vi "SPM Pump v0.5.vi"(0 "Termination char\n(0xA = '\\n' = LF)\n(0xD = '\\r' = CR)":u8=13 format="%.0x", 1 "Enable Termination\nChar (T)":bool=TRUE, 2 "Timeout (ms)":u32=10000, 3 "Serial Settings:Serial End Mode for Reads":u16(ring)=2 items=["None", "LastBit", "TermChar"], 4 "byte count":u32=64, 5 "Delay before read (ms)":u32=1000, 6 "Time <input>":dbl, 7 "error in (no error)":errorcluster, 8 "Serial port input":string="/1ZR", 9 "VISA resource name":refnum<visa-resource-name>="COM6", 10 "parity":u16(ring) items=["None", "Odd", "Even", "Mark", "Space"], 11 "baud rate":u32=9600, 12 "stop bits":u16(ring)=10 items=["1.0"=10, "1.5"=15, "2.0"=20], 13 "data bits":u16=8 min=5 max=8 step=1, 14 "flow control":u16(ring) items=["None"=0, "XON/XOFF"=1, "RTS/CTS"=2, "DTR/DSR"=4], 15 "Time units <input>":string) -> (16 "Input command":string, 18 "Pump status":string, 20 "Start speed":i32, 21 "Maximal speed":i32, 22 "Cutoff speed":i32, 23 "Valve position":i32, 24 "Absolute plunger position":i32, 25 "Actual plunger position":i32, 26 "Serial port":string, 27 "error out":errorcluster)   [LabVIEW 2016]
doc: "The Basic Serial Read and Write example performs a Serial Port Read, a Serial Port Write, or a combination of these actions. The user selects the actions (read or write) on the front panel. If both are selected, the VI will write the data first, read data, and then close the VISA session that is opened to the port. This VI will wait until the specified number of bytes is received at the port. Only the number of bytes specified will be read.\n\nINSTRUCTIONS:\n1) Select the serial resource and configuration parameters (baud rate, data bits, parity, stop bits, flow control).\n2) Select the operations to be performed. \n3) Connect the serial port to your device. If no device is available, perform a loopback test by doing one of the following. Short pins 2 and 3 on a RS-232 cable or short pin 4 to pin 8 and pin 5 to pin 9 on a RS-485/422 cable. \n4) Run the VI to see the data read. (The \"read string\" will match the \"string to write\" if a loopback test was performed.)\n\nNote: The parameters set for the serial port must match the parameters of the connected instrument or device. In this example, the bytes to read parameter specifies the number of bytes that the serial port reads. If there were more bytes at the port than the number specified in bytes to read, those bytes would not be read. Also, if you specify to read more bytes than the number of bytes actually read, you might receive a timeout error message.\n\nOn the block diagram, the Configure Serial Port VI sets the configuration parameters. The front panel displays the controls used to configure the basic parameters, such as baud rate, data bits, and parity. Constants configure the other parameters the user probably does not need set. After the VISA Configure Serial Port VI opens the VISA session and configures the port, the VI passes the VISA resource name to other VIs that perform operations on that VISA resource. The VISA Write function sends a command to the serial device and the VISA Read function returns data based on the command. The VISA Close function then closes the reference to the serial device. It is important to close the reference; otherwise communication through with that port through protocols other than VISA might not be possible."
panel:
  # "Select the serial resource and the operations (Read, Write, or both) to be performed.  If both are selected, the VI will write the data first, read data and then close the VISA session that is opened to the port.  This VI will wait until the specified number of bytes is received at the port. Only the number of bytes specified will be read."
  # "For additional information select File >> VI Properties >> Documentation"
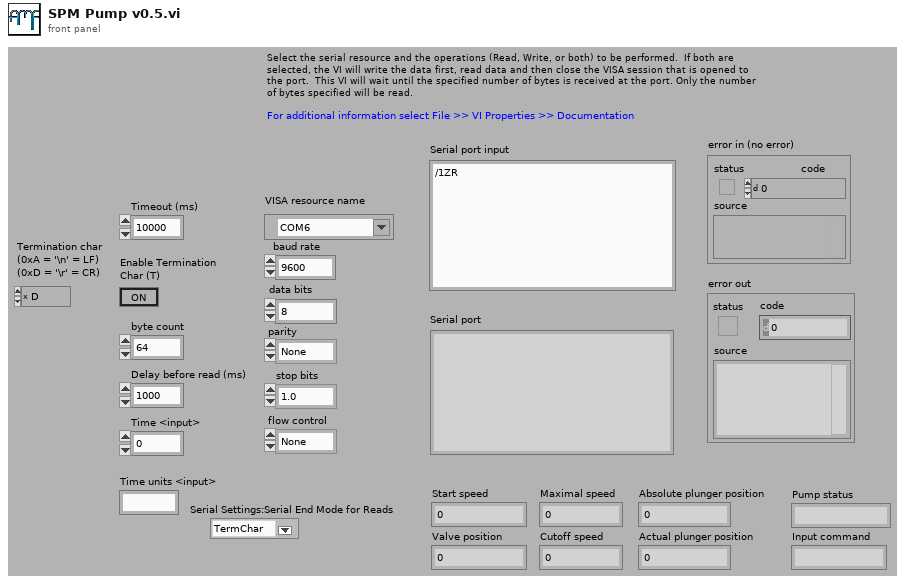
[diagram p1: front panel]
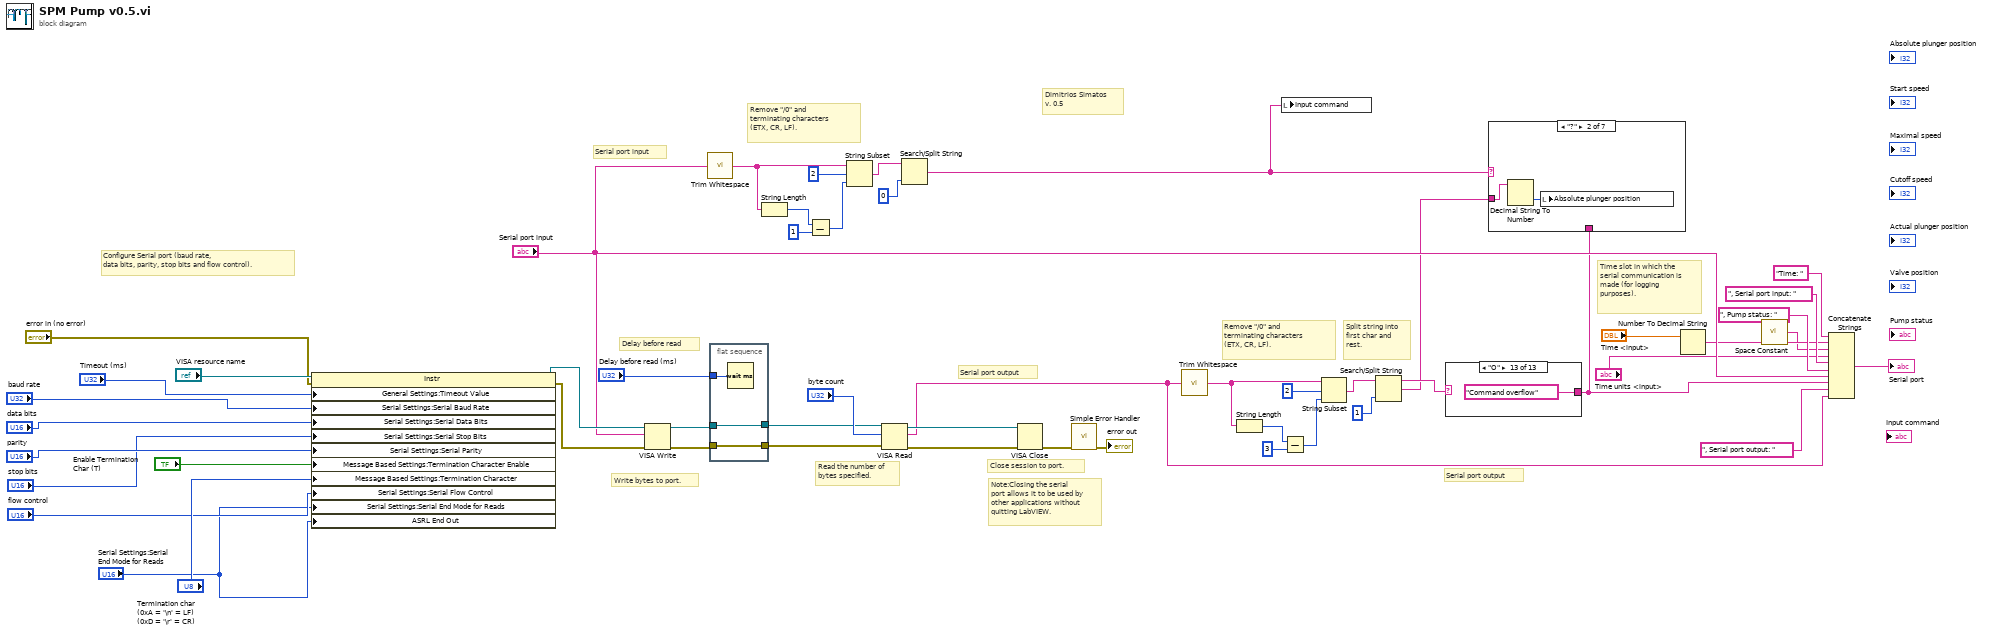
[diagram p0: block diagram]
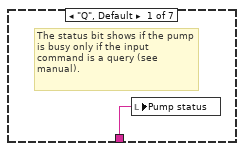
[diagram p2: hidden frame]
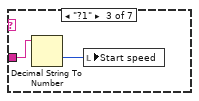
[diagram p3: hidden frame]
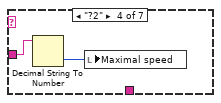
[diagram p4: hidden frame]
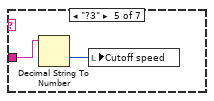
[diagram p5: hidden frame]
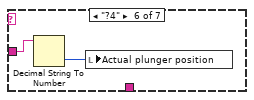
[diagram p6: hidden frame]
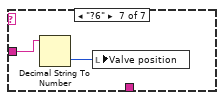
[diagram p7: hidden frame]
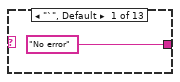
[diagram p8: hidden frame]
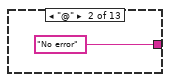
[diagram p9: hidden frame]
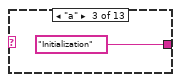
[diagram p10: hidden frame]
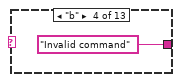
[diagram p11: hidden frame]
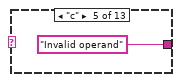
[diagram p12: hidden frame]
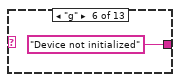
[diagram p13: hidden frame]
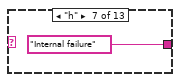
[diagram p14: hidden frame]
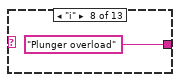
[diagram p15: hidden frame]
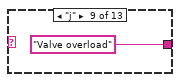
[diagram p16: hidden frame]
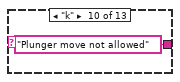
[diagram p17: hidden frame]
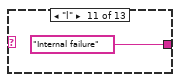
[diagram p18: hidden frame]
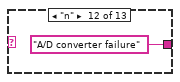
[diagram p19: hidden frame]
diagram:
  # "Serial port input"
  # "Remove \"/0\" and terminating characters (ETX, CR, LF)."
  # "Serial port output"
  # "Serial port output"
  # "Time slot in which the serial communication is made (for logging purposes)."
  # "Split string into first char and rest."
  # "Remove \"/0\" and terminating characters (ETX, CR, LF)."
  # "Delay before read"
  # "Dimitrios Simatos\nv. 0.5"
  # "Read the number of bytes specified."
  # "Write bytes to port."
  # "Note:Closing the serial port allows it to be used by other applications without\nquitting LabVIEW."
  # "Configure Serial port (baud rate,\ndata bits, parity, stop bits and flow control)."
  # "Close session to port."
  n1 = property class="Instr"(reference="VISA resource name", error in="error in (no error)", "General Settings:Timeout Value"="Timeout (ms)", "Serial Settings:Serial Baud Rate"="baud rate", "Serial Settings:Serial Data Bits"="data bits", "Serial Settings:Serial Stop Bits"="stop bits", "Serial Settings:Serial Parity"="parity", "Message Based Settings:Termination Character Enable"="Enable Termination\nChar (T)", "Message Based Settings:Termination Character"="Termination char\n(0xA = '\\n' = LF)\n(0xD = '\\r' = CR)", "Serial Settings:Serial Flow Control"="flow control", "Serial Settings:Serial End Mode for Reads"="Serial Settings:Serial End Mode for Reads", "ASRL End Out"="Serial Settings:Serial End Mode for Reads") -> (reference out=w39:refnum<visa-resource-name>, error out=w38:errorcluster)
  n2 = VISA Write(VISA resource name=w39, write buffer="Serial port input", error in (no error)=w38) -> (VISA resource name out=w34:refnum<visa-resource-name>, error out=w33:errorcluster)  [unwired: 1 out]
  n3 = call <vilib>:"Trim Whitespace.vi"("string"="Serial port input") -> ("trimmed string"=w12:string)  [unwired: 1 in]
  n4 = flat-sequence {
    tunnel: w33 -> [w54]
    tunnel: [w54] -> w32
    tunnel: w34 -> [w53]
    tunnel: [w53] -> w31
    tunnel: "Delay before read (ms)" -> [w55]
    frame #0 {
      n5 = Wait (ms)(milliseconds to wait=w55) -> ()  [unwired: 1 out]
    }
  }
  n6 = String Length(string=w12) -> (length=w16:i32)
  n7 = Subtract(x=w16, y=1) -> (x-y=w15:i32)
  n8 = String Subset(string=w12, offset (0)=2, length (rest)=w15) -> (substring=w9:string)
  n9 = VISA Read(VISA resource name=w31, byte count="byte count", error in (no error)=w32) -> (VISA resource name out=w51:refnum<visa-resource-name>, read buffer=w18:string, error out=w52:errorcluster)  [unwired: 1 out]
  n10 = Search/Split String(string=w9, offset (0)=0) -> (match + rest of string=w1:string)  [unwired: 1 in, 2 out]
  n11 = VISA Close(VISA resource name=w51, error in (no error)=w52) -> (error out=w50:errorcluster)
  n12 = call <vilib>:"Simple Error Handler.vi"("error in (no error)"=w50) -> ("error out"=→"error out":errorcluster)  [unwired: 4 in, 4 out]
  n13 = call <vilib>:"Trim Whitespace.vi"("string"=w18) -> ("trimmed string"=w25:string)  [unwired: 1 in]
  n14 = String Length(string=w25) -> (length=w29:i32)
  n15 = local write "Input command"(w1) -> ()
  n16 = Subtract(x=w29, y=3) -> (x-y=w28:i32)
  n17 = String Subset(string=w25, offset (0)=2, length (rest)=w28) -> (substring=w24:string)
  n18 = Search/Split String(string=w24, offset (0)=1) -> (substring before match=w22:string, match + rest of string=w8:string)  [unwired: 1 in, 1 out]
  n19 = case shown="\"O\"" w22 {
    tunnel: ["No error" "No error" "Initialization" "Invalid command" "Invalid operand" "Device not initialized" "Internal failure" "Plunger overload" "Valve overload" "Plunger move not allowed" "Internal failure" "A/D converter failure" "Command overflow"] -> w7
    frame "`", Default {
    }
    frame "@" {
    }
    frame "a" {
    }
    frame "b" {
    }
    frame "c" {
    }
    frame "g" {
    }
    frame "h" {
    }
    frame "i" {
    }
    frame "j" {
    }
    frame "k" {
    }
    frame "l" {
    }
    frame "n" {
    }
    frame "O" {
    }
  }
  n20 = case shown="\"?\"" w1 {
    tunnel: w8 -> [_ w70 w72 w75 w76 w79 w81]
    tunnel: w7 -> [w69 _ _ _ _ _ _]
    frame "Q", Default {
      # "The status bit shows if the pump is busy only if the input command is a query (see manual)."
      n21 = local write "Pump status"(w69) -> ()
    }
    frame "?" {
      n22 = Decimal String To Number(string=w70) -> (number=w71:i32)  [unwired: 2 in, 1 out]
      n23 = local write "Absolute plunger position"(w71) -> ()
    }
    frame "?1" {
      n24 = Decimal String To Number(string=w72) -> (number=w73:i32)  [unwired: 2 in, 1 out]
      n25 = local write "Start speed"(w73) -> ()
    }
    frame "?2" {
      n26 = Decimal String To Number(string=w75) -> (number=w74:i32)  [unwired: 2 in, 1 out]
      n27 = local write "Maximal speed"(w74) -> ()
    }
    frame "?3" {
      n28 = Decimal String To Number(string=w76) -> (number=w77:i32)  [unwired: 2 in, 1 out]
      n29 = local write "Cutoff speed"(w77) -> ()
    }
    frame "?4" {
      n30 = Decimal String To Number(string=w79) -> (number=w78:i32)  [unwired: 2 in, 1 out]
      n31 = local write "Actual plunger position"(w78) -> ()
    }
    frame "?6" {
      n32 = Decimal String To Number(string=w81) -> (number=w80:i32)  [unwired: 2 in, 1 out]
      n33 = local write "Valve position"(w80) -> ()
    }
  }
  n34 = Number To Decimal String(number="Time <input>") -> (decimal integer string=w4:string)  [unwired: 1 in]
  n35 = call <vilib>:"Space Constant.vi"() -> ("String"=w2:string)
  n36 = Concatenate Strings("Time: ", w4, w2, "Time units <input>", ", Serial port input: ", "Serial port input", ", Pump status: ", w7, ", Serial port output: ", w18) -> (→"Serial port":string)
